vi "WS_RS485ETH_get.vi"(5 "param_num":string="740", 7 "address":string="022", 8 "error in":errorcluster, 9 "data":string="=?", 10 "data_length":string="2", 11 "conn_id_in":refnum<k5>) -> (0 "error out":errorcluster, 2 "response":string, 3 "conn_id_out":refnum<k5>, 4 "status":bool)   [LabVIEW 2019]
panel:
  in  "timeout ms":i32=1000
  out "command":string
  in  "action":string="00"
  # "00 = data request, 10 = control command"
  # "3 digits"
  # "3 digits"
  # "2 digits"
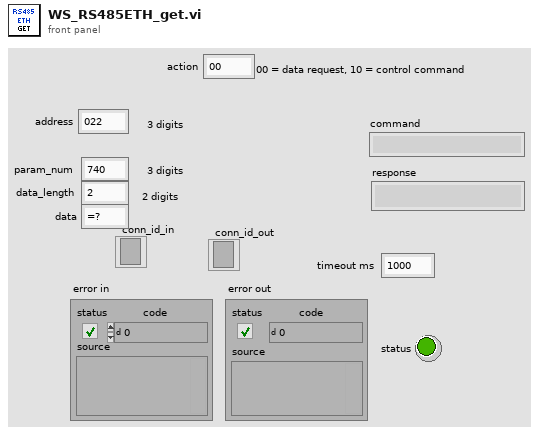
[diagram p1: front panel]
types:
  T1 = enum16{"Standard", "Buffered", "CRLF", "Immediate"}
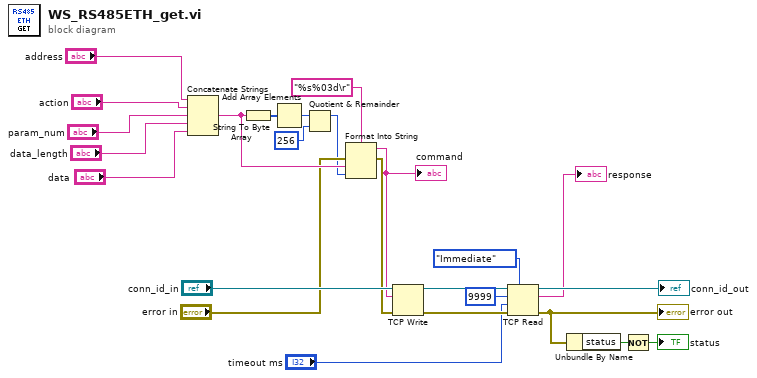
[diagram p0: block diagram]
diagram:
  n1 = Concatenate Strings("address", "action", "param_num", "data_length", "data") -> (w6:string)
  n2 = String To Byte Array(string=w6) -> (unsigned byte array=w10:u8[])
  n3 = Add Array Elements(numeric array=w10) -> (sum=w8:u8)
  n4 = Quotient & Remainder(x=w8, y=u64 256) -> (x-y*floor(x/y)=w1:u64)  [unwired: 1 out]
  n5 = Format Into String(format string="%s%03d\r", error in="error in", w6, w1) -> (resulting string=w5:string, error out=w3:errorcluster)  [unwired: 1 in]
  "command" <- w5
  n6 = TCP Write(connection ID="conn_id_in", data in=w5, error in (no error)=w3) -> (connection ID out=w24:refnum<k5>, error out=w25:errorcluster)  [unwired: 1 in, 1 out]
  n7 = TCP Read(connection ID=w24, bytes to read=9999, error in (no error)=w25, 7:T1."Immediate" ("mode (standard)"), 9:"timeout ms") -> (connection ID out=→"conn_id_out":refnum<k5>, data out=→"response":string, error out=w19:errorcluster)
  "error out" <- w19
  n8 = Unbundle By Name(w19) -> ("status"=w18:bool)
  n9 = Not(x=w18) -> (.not. x?=→"status":bool)
